vi "UHR-Fleezers Control (host) - 16.2.2v2.vi"() -> ()   [LabVIEW 2014] (continued)
  in  "Limits Enable":bool=TRUE caption="Enable"
  out "AI labels":string[](array[string])=["T1 Y", "T1 X", "T1 Sum", "T2 Y", "T2 X", "T2 Sum", "T1 FB X", "T1 FB Sum", "T2 FB X", "T2 FB Sum", "PSD Y", "PSD X", "PSD Y Sum"]
  in  "Save Trap Pos. Data":bool=TRUE
  in  "Lower Ch. Cap.":bool
  in  "Top 3 Harvard Syringe Pump Serial Port":refnum<visa-resource-name>="Top-Pump3-COM4"
  out "Database link":path
  out "connection reference":T19
  out "FPGA error out":errorcluster
  out "Trigger Signal":dbl[](graph)
  in  "Fish mask thresh":dbl=0.5
  in  "Normal (on) or masked test (off)":bool=TRUE
  in  "Stop F (pN) (mask)":dbl=1.0
  in  "Osc. freq. (Hz)":dbl=0.25
  in  "Trap shift\nmethod":bool=TRUE
  in  "Pause rotation":bool
  out "Waveform Chart":dbl(graph)
  in  "Trap 2 phase shift (deg)":dbl caption="Fixed phase shift (deg)"
  in  "Radius (MHz)":dbl=2.0 min=0.0 max=10.0 step=0.1
  out "Trap trajectories":cluster{dbl[], dbl[]}[](graph)
  in  "Move in a Circle":bool
  in  "Center Y Frequency (MHz)":dbl=31.0
  in  "Stop Moving":bool
  in  "2D Motion Frequency (Hz)":dbl=0.25
  in  "2D Motion Trap Separation (MHz)":dbl=0.75 caption="Fixed distance (MHz)" min=0.0 max=10.0 step=0.1
  in  "Time step (ms)":i64=10
  in  "N steps then stop":i32
  in  "Back to start on finish?":bool=TRUE
  in  "Counterclockwise/Clockwise":bool
  out "Trap 1 sum mean":dbl format="%0.2f"
  out "Trap 2 sum mean":dbl format="%0.2f"
  in  "index 1":i32=3
  in  "index 2":i32
  in  "test":bool
  in  "Reset graph":bool
  in  "N steps to plot":i32=1000
  out "Waveform Graph 2":waveform(dbl)(graph)
  in  "Offset 2":dbl
  in  "mult x":dbl
  in  "Offset":dbl
  out "N data samples":dbl
  out "Initial buffer time (s)":dbl
  in  "N initial buffer elements":u16=5000
  in  "Sound ON":bool
  in  "Carrier Frequency (Hz)":dbl=300.0
  in  "number of samples/ch":i32=100000
  in  "sample mode":T20=1 items=["Finite Samples", "Continuous Samples"]
  in  "device ID":u32
  in  "sound format":T21={"sample rate (S/s)"=22050.0, "number of channels"=2, "bits per sample"=16}
  in  "Volume":dbl=1.0 format="%0.2p"
  in  "interpolation mode":u16(ring)=1 items=["coerce", "linear", "spline", "FIR filter"]
  in  "tone or data":bool
  in  "Data channel to sound":i32
  in  "Base N trap periods":u32=50
  in  "Period scale factor":dbl=4.0
  in  "Trap osc amp (MHz)":dbl=1.0
  in  "Osc trap cont.":bool
  in  "Osc traps":bool
  out "Trap OSC Period (s)":dbl
  out "Writing waveform to fpga memory":bool
  in  "Save trap pos with cal":bool=TRUE
  in  "T1 Osc Enable":bool=TRUE
  in  "T2 Osc Enable":bool=TRUE
  out "DMA remainder":u64
  out "(total save/100) /osc period remainder":u32
  out "Total save/100 remainder":u32
  out "N osc/ (total save/100)":u64
  out "N osc / DMA":u64
  out "N trap osc periods per save":u64
  out "N trap osc periods per save remainder":u64
  in  "Command":string
  out "Reply":string
  in  "Send Command":bool
  out "Preamp Error Out":errorcluster
  in  "Gain Mode":string(combo)="0"
  in  "Invert Signal":bool
  in  "Sensitivity":string(combo)="0"
  in  "Offset Current Sign":bool=TRUE
  in  "Offset Current Value":string(combo)
  in  "Offset Current":bool
  in  "Bias Voltage":bool
  in  "Bias Voltage (mV)":i32
  in  "Filter Type":string(combo)="4"
  in  "Lowpass 3dB Point":string(combo)="6"
  in  "Highpass 3dB Point":string(combo)
  in  "Filter Reset":bool
  out "Command Sent":string
  out "Gain":string(combo)="0"
  # "X"
  # "Y"
  # "APD counting rates"
  # "External fluorescence triggering tests:"
  # "After"
  # "During"
  # "Trap On?"
  # "BD Flow ON?"
  # "Samp Flow ON?"
  # "Trap Trig. Fl.?"
  # "Zero It"
  # "Floor it\n(e.g., hp unwinding)"
  # "1"
  # "2"
  # "Fl. Down"
  # "Fl. Up"
  # "Slowly scan trap from current position to an offset.\nMake range negative to go backwards.\nUses rough Windows timing. \nUpdates trap Delta. \nCan cancel and traps will stay at last position."
  # "Trap Display:"
  # "APD Display:"
  # "Lifetime measurements cannot be make\nat the same time as recording trap positions.\nSo constant force feedback measurements can't be done\n(though constant force can be maintained, just not saved).\nTrap positions also can't be used to do dynamic offset subtraction\n(using the offset curve)."
  # "FPGA DAQ"
  # "Data Saving"
  # "Trap Manipulation"
  # "Bead Calibration"
  # "Fine Motor Control"
  # "Bottom Pump (#1)"
  # "Central Sample Channels"
  # "Top Pump (#3)"
  # "Rate param is ul/h\nVolume param is ul"
  # "Chemyx Pump 2"
  # "Units: \n1 = ml/m\n2 = ml/h\n3 = ul/m\n4 = ul/h"
  # "Some timing delay counts"
  # "Oscillate Set 1 freq. (debugging)"
  # "If using 2nd RF synth board to control green:\nThen small change in FPGA code to make sets 1 and 2\ncorrespond always to board F1 and F2 so green\ndigital out switches between set 1 and 2 frequencies. \nNo third period. \nSet freq for sets 1 and 3 is zero, set 2 is 80 MHz.\nSet amplitude of all three sets to the same value - no feedback yet."
  # "BD 1"
  # "BD 2"
  # "For trap X control"
  # "For green AOM or trap Y control"
  # "Trap interlacing RF phase control"
  # "Phase control methods:\n0 = no phase control\n1 = offset increments each trap cycle by values below\n2 = offset increment increases by increment factor each cycle\n3 = random phase (no parameters to set)"
  # "X"
  # "Y"
  # "Only runs at startup. As of 161102, 30% out gives saturated max AOM out. Amp control is 12 bits, so this max corresponds to ~1300."
  # "14-bit phase number, i.e., 0 to 16383 (2^14) covers full 2*pi phase."
  # "AOD Raster Scan"
  # "Approx. trap separations"
  # "X"
  # "Y"
  # "FPGA\nreading"
  # "DMA\ntransfer"
  # "APD Integration Loop"
  # "APD Gates"
  # "Controls below are for integration occuring right after DMA transfer from FPGA.\nAffects all labview analysis and plotting of fluorescence. \nBUT does not affect data saving. Data is saved at full FPGA integration timing."
  # "APD 2 (Cy5)"
  # "APD 3 (Cy2)"
  # "This needs to be an integer to match trap and fluorescence data transfer timing."
  # "APD 1 (Cy3)"
  # "X"
  # "2D"
  # "Y"
  # "1D"
  # "For producing an anlalog output signal for APDs that can be connected to an oscilloscope and used for alignment within the trap room.\n\nPay attention to FPGA integration time. Needs to be high enough to produce a good signal for each time point. So for a 10 kHz mean fluorescence signal, try 10 ms integration, which would give 100 photons per time point on average."
  # "To switch the excitation laser\nintensity setpoint for each bead pair\n(switches when fishing begins)"
  # "Digital Out Control"
  # "Analog Out Control (Feedback Loop)"
  # "Laser Intensity Analog Input"
  # "Operational note:\n\nUse the digital out control to adjust red laser\ntiming (fine tuning).\n\nAt the moment, the red laser analog out\ncontrol timing is identical and set by green \nlaser AO timing (in the same loop).  Otherwise\nyou can not get synchronous timing with the\ncurrent AO expansion board.\n\nSimilarly, the AI measurement is also \nsimultaneous for all three lasers (for the same\nreason).\n\nThese controls are kept for possible future\nuse."
  # "Analog Out Control (Feedback Loop)"
  # "Digital Out Control"
  # "Laser Intensity Analog Input"
  # "Operational note:\n\nThe AI measurement is simultaneous for all three lasers\n(see red laser note).\n\nThese controls are kept for possible future use."
  # "Analog Out Control (Feedback Loop)"
  # "Laser Intensity Analog Input"
  # "Digital Out Control"
  # "Only initial FIFO depth is set - cannot change while running instrument (will give buffer status error)"
  # "Total AI Rates (NOT rates/trap)"
  # "(Samples/trap x Trap Sets)"
  # "(Samples/channel x\n8 if averaging (8 channels)\n4 if no averaging)"
  # "Trap 1"
  # "Trap 2"
  # "Flour./Trap 3"
  # "External Video Window"
  # "3: IR LED\n2: Blue LED"
  # "MCL Position Debugging"
  # "Temporary Control Storage\n(these used to be somewhere else, still want to keep them)"
  # "Database config"
  # "Y"
  # "X"
  # "Trap Position Difference Limits"
  # "Start trapping above center (> center MHz)\n\nNegative trap separation means trap 2 follows\n(starts to the right)"
  # "Initialization"
  # "Radius initially determined by center\nand current location (then can be changed)"
  # "Active (oscillating) trap calibration:"
  # "All these remainders\nshould be 0."
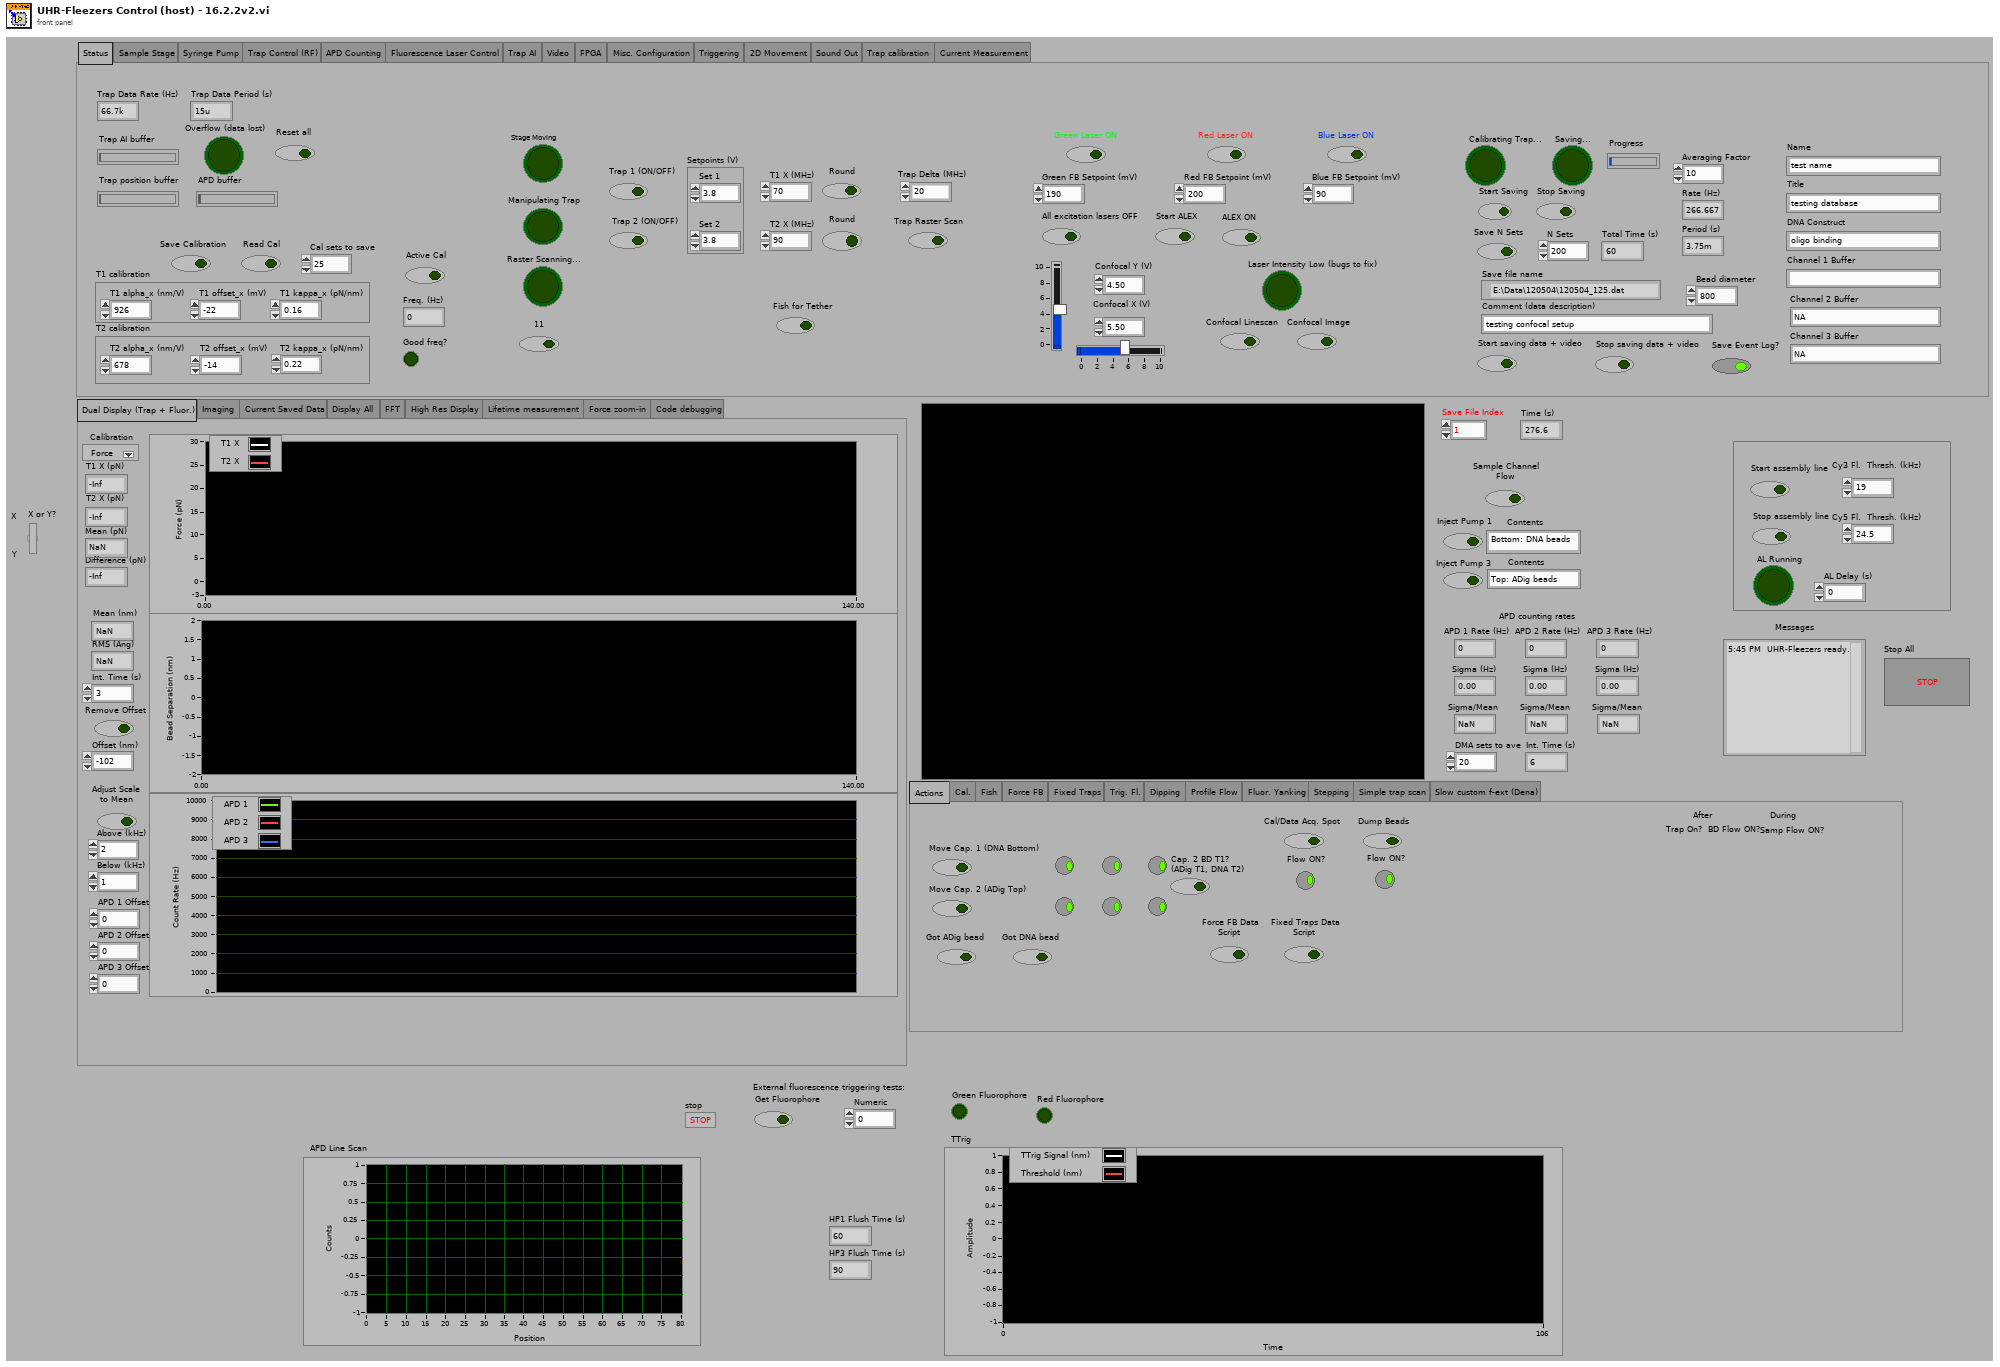
[diagram p1: front panel]
types:
  T1 = enum32{"Actions", "Cal.", "Fish", "Force FB", "Fixed Traps", "Trig. Fl.", "Dipping", "Profile Flow", "Fluor. Yanking", "Stepping", "Simple trap scan", "Slow custom f-ext (Dena)"}
  T2 = typedef "IMAQ Image.ctl" = refnum<image>
  T3 = enum32{"Dual Display (Trap + Fluor.)", "Imaging", "Current Saved Data", "Display All", "FFT", "High Res Display", "Lifetime measurement", "Force zoom-in", "Code debugging"}
  T4 = enum32{"Status", "Sample Stage", "Syringe Pump", "Trap Control (RF)", "APD Counting", "Fluorescence Laser Control", "Trap AI", "Video", "FPGA", "Misc. Configuration", "Triggering", "2D Movement", "Sound Out", "Trap calibration", "Current Measurement"}
  T5 = cluster{"T2 alpha_x (nm/V)":dbl, "T2 offset_x (mV)":dbl, "T2 kappa_x (pN/nm)":dbl}
  T6 = cluster{"T1 alpha_x (nm/V)":dbl, "T1 offset_x (mV)":dbl, "T1 kappa_x (pN/nm)":dbl}
  T7 = cluster{"Pump 1":cluster{"Diameter (mm)":dbl, "Units":dbl, "Volume":dbl, "Rate":dbl}, "Pump 2":cluster{"Diameter (mm)":dbl, "Units":dbl, "Volume":dbl, "Rate":dbl}, "Pump 3":cluster{"Diameter (mm)":dbl, "Units":dbl, "Volume":dbl, "Rate":dbl}}
  T8 = enum32{"IR Laser Interlacing (Direct RF Board Control Method)", "AOD Raster Scan", "Feedback on Trap Intensity", "Feedback on Trap Position"}
  T9 = typedef "LVPoint32TypeDef.ctl" = cluster{"Horizontal":i32, "Vertical":i32}
  T10 = cluster{"Scan Range AOD (nm) 2":dbl, "Step Size AOD (nm) 2":dbl, "Scan Speed AOD (nm/s) 2":dbl, "Number of scans (AOD) 2":u16, "Label":string}[]
  T11 = cluster{"proportional gain (Kc)":i16, "integral gain (Kc*Ts/Ti)":i16, "derivative gain (Kc*Td/Ts)":i16}
  T12 = cluster{"Trap 1":fxp<+/-,16,1>, "Trap 2":fxp<+/-,16,1>}
  T13 = cluster{"proportional gain (Kc)":fxp<+/-,16,8>, "integral gain (Kc*Ts/Ti)":fxp<+/-,16,8>, "derivative gain (Kc*Td/Ts)":fxp<+/-,16,8>}
  T14 = cluster{"output high":fxp<+/-,16,1>, "output low":fxp<+/-,16,1>}
  T15 = cluster{"Set 1":fxp<+/-,16,1>, "Set 2":fxp<+/-,16,1>}
  T16 = enum32{"Main Controls", "Green laser (532 nm)", "Red laser (633 nm)", "Blue laser (473 nm)"}
  T17 = cluster{"Set 1":bool, "Set 2":bool, "Set 3":bool}
  T18 = typedef "LVMinMaxIncTypeDef.ctl" = cluster{"Minimum":dbl, "Maximum":dbl, "Increment":dbl}
  T19 = typedef "NI_Database_API.lvlib/Conn ObjectReference.ctl" = refnum<k1>
  T20 = typedef "Sampling Mode.ctl" = i32
  T21 = typedef "Sound Data Format.ctl" = cluster{"sample rate (S/s)":dbl, "number of channels":i32, "bits per sample":i32}
  T22 = typedef "Image Type" = u32
  T23 = typedef "nirio_resource_hc.ctl" = tag
  T24 = typedef "openfpgaref.initrf.ctl" = refnum<k20>
  T25 = typedef "openfpgaref.8.6.ctl" = refnum<k20>
  T26 = enum16{"empty", "write", "read oldest (queue)", "read newest (stack)", "read all"}
  T27 = cluster{"New Image":T2, "New Image":T2, "New Image":T2, "New Image":T2, "New Image":T2}
  T28 = typedef "XDNodeRunTimeDep.lvlib/timing_clust.ctl" = cluster{"Expected End [f-1]":u64, "Actual End [f-1]":u64, "Finished Late? [f-1]":bool, "Expected End [i-1]":u64, "Actual End [i-1]":u64, "Finished Late? [i-1]":bool, "Expected Start [i]":u64, "Actual Start [i]":u64, "Expected Start [f]":u64, "Actual Start [f]":u64, "Source Name":string, "Structure Name":string, "Period":i64, "Deadline":i64, "Offset":i64, "Start":i64, "Priority":i32, "Timeout":i32, "Mode":T29, "Wakeup Reason":T30, "Error":errorcluster, "Source Type":string, "Secondary Source Type":string, "Global End Time":u64, "Global Start Time":u64, "Frame Duration":u64, "Iteration Duration":u64, "Assigned CPU":i32, "I/O Scan Engine Mode":u32}
  T29 = typedef "XDNodeRunTimeDep.lvlib/nitl_modes.ctl" = enum32{"No Change", "Process missed periods, maintain original phase", "Discard missed periods, maintain original phase", "Process missed periods, ignore original phase", "Discard missed periods, ignore original phase"}
  T30 = typedef "XDNodeRunTimeDep.lvlib/wakeup.ctl" = enum32{"Normal", "Aborted", "Asynchronous wakeup", "Timing source error", "Timed loop error", "Timeout"}
  T31 = enum32{"Status", "Sample Stage", "Syringe Pump", "Trap Control (RF)", "APD Counting", "Fluorescence Laser Control", "Trap AI", "Video", "FPGA"}
  T32 = enum32{"Status", "Sample Stage", "Syringe Pump", "Trap Control (RF)", "APD Counting", "Fluorescence Laser Control", "Trap AI", "Video", "FPGA", "Misc. Configuration"}
  T33 = enum32{"Actions", "Cal.", "Fish", "Force FB", "Fixed Traps", "Trig. Fl.", "Dipping", "Profile Flow", "Fluor. Yanking", "Stepping"}
  T34 = enum16{"big-endian, network order", "native, host order", "little-endian"}
  T35 = enum16{"open", "replace", "create", "open or create", "replace or create", "replace or create with confirmation"}
  T36 = cluster{"Left":i32, "Top":i32, "Width":u32, "Height":u32}
  T37 = cluster{cluster{"Left":i32, "Top":i32, "Width":u32, "Height":u32}}[]
  T38 = cluster{"Scan Range AOD (nm) 2":dbl, "Step Size AOD (nm) 2":dbl, "Scan Speed AOD (nm/s) 2":dbl, "Number of scans (AOD) 2":u16, "Label":string}
  T39 = cluster{"[0]":dbl, "[1]":dbl, "[2]":dbl, "[3]":dbl, "[4]":dbl, "[5]":dbl}
  T40 = cluster{"Diameter (mm)":dbl, "Units":dbl, "Volume":dbl, "Rate":dbl}
  T41 = enum32{"setting", "request", "request control", "info", "statistics", "system settings", "I/O sub system", "HRT control", "camera descriptions", "device specific data", "event sub system settings", "event sub system results", "image memory manager"}
  T42 = typedef "IMAQ AVI2 Refnum.ctl" = refnum<k20>
  T43 = typedef "imagedata.ctl" = cluster{"image type":i32, "image depth":i32, "image":u8[], "mask":u8[], "colors":u32[], "Rectangle":cluster{"left":i16, "top":i16, "right":i16, "bottom":i16}}
  T44 = typedef "Sound Output Task ID.ctl" = u32
  T45 = enum32{"Normal Display", "Dual Display (APD)", "FFT", "High Res Display"}
  T46 = cluster{"Origin Pixel":cluster{"X":sgl, "Y":sgl}, "Angle Relative to Horizontal (deg)":sgl, "Axis Reference":u32}
  T47 = typedef "Simple Grid Descriptor" = cluster{"X Step":sgl, "Y Step":sgl, "Unit":T48}
  T48 = typedef "Image Unit" = enum32{"Undefined", "Angström", "Micrometer", "Millimeter", "Centimeter", "Meter", "Kilometer", "Microinch", "Inch", "Feet", "Nautical miles", "Standard miles", "Steps"}
  T49 = enum32{"Dual Display (Trap + Fluor.)", "Imaging", "Current Saved Data", "Display All", "FFT", "High Res Display"}
  T50 = cluster{"averaging mode":u16, "weighting mode":u16, "number of averages":u32}
  T51 = cluster{"dB On (F)":bool, "unwrap phase (F)":bool, "convert to degree (F)":bool}
  T52 = cluster{"Array Out":dbl[], "Array Out":dbl[], "Array Out":dbl[]}
  T53 = cluster{string, string, string, string, string, string, string, string}
  T54 = cluster{string, string, string, string, string, string, string, string, string, string, string, string}
  T55 = cluster{string, string, string, string, string, string, string, string, string, string, string, string, string}
  T56 = cluster{string, string, string, string, string, string, string, string, string, string, string, string, string, string}
  T57 = cluster{"BD 1 Frequency 1 (MHz)":dbl, "BD 1 Frequency 2 (MHz)":dbl}
  T58 = cluster{"f0":dbl, "df":dbl, "magnitude":dbl[]}[][]
  T59 = cluster{"Comment (data description)":string, "Channel 1 Buffer":string, "Channel 2 Buffer":string, "Channel 3 Buffer":string, "Title":string, "DNA Construct":string, "Bead diameter":dbl, "Name":string}
diagram:
  w7 = u16 20 items=["1.0"=10, "1.5"=15, "2.0"=20] ("stop bits (10: 1 bit)")
  w19 = u16 20 items=["1.0"=10, "1.5"=15, "2.0"=20] ("stop bits (10: 1 bit)")
  w43 = u16 10 items=["1.0"=10, "1.5"=15, "2.0"=20] ("stop bits (10: 1 bit)")
  w56 = u16 20 items=["1.0"=10, "1.5"=15, "2.0"=20] ("stop bits (10: 1 bit)")
  w58 = u16 20 items=["1.0"=10, "1.5"=15, "2.0"=20] ("stop bits (10: 1 bit)")
  w65 = u16 20 items=["1.0"=10, "1.5"=15, "2.0"=20] ("stop bits (10: 1 bit)")
  w48 = T22 2 items=["Grayscale (U8)", "Grayscale (I16)", "Grayscale (SGL)", "Complex (CSG)", "RGB (U32)", "HSL (U32)", "RGB (U64)", "Grayscale (U16)"] ("Image Type")
  # "n samples needed for data"
  # "Settings to help prevent AOM/D damage"
  # "Bottom 1 Harvard"
  # "Top 3 Harvard"
  # "Center Harvard"
  # "Bottom 1 Harvard"
  # "Top 3 Harvard"
  # "Center Harvard"
  n1 = flat-sequence {
    tunnel: [w107] -> w3
    tunnel: [w103] -> w2
    tunnel: w3 -> [w115]
    tunnel: w2 -> [_]
    tunnel: [w110] -> w1
    frame #0 {
      w107 = T23 "750kHzDAQ" ("resource name")
      # "DAQ card ID"
      # "First run the RF synth board initialization fpga code.\n\nThis fpga code essentially enables communication with the RF board using the automatic udclk setting. After running the host initialization vi, the RF boards are fully setup and ready to interlace using the external udclk control. The next fpga code runs the main interlacing instrument methods.\n\nThis host code should run the init bitfile:\n\n'UHR-FleezersInst_FPGATarget_intitializeRFsyn_v1'"
      n2 = xnode "Open FPGA VI Reference"("resource name"=w107) -> ("FPGA VI Reference Out"=w106:refnum<k20>)  [unwired: 1 in, 1 out]
      n3 = xnode "Invoke Method"("FPGA VI Reference In"=w106) -> ("FPGA VI Reference Out"=w100:refnum<k20>, "error out"=w99:errorcluster)  [unwired: 1 in]
      n4 = xnode "Invoke Method"("FPGA VI Reference In"=w100, "error in"=w99) -> ("FPGA VI Reference Out"=w102:refnum<k20>, "error out"=w101:errorcluster)  [unwired: 1 in]
      n5 = call "Initialize RF boards - with FPGA init only vi v1.vi"("error in"=w101, "FPGA Interface"=w102) -> ("error out"=w104:errorcluster, "FPGA Interface 2"=w105:T24)
      n6 = xnode "Close FPGA VI Reference"("FPGA VI Reference In"=w105, "error in"=w104) -> ("error out"=w103:errorcluster)
    }
    frame #1 {
      w108 = TRUE ("PMODE")
      # "Have to set parallel mode and read to high again (they default to low in the FPGA code)"
      # "Then switch to the main fpga code to run the instrument (interlacing fpga code).\n\nThis host code should run the bitfile:\n\n'UHR-FleezersInst_FPGATarget_UHR-Fleezers_main_16.2.1_v3'"
      # "Reset the DAQ card."
      n7 = xnode "Open FPGA VI Reference"("resource name"=w115) -> ("FPGA VI Reference Out"=w114:T25, "error out"=w113:errorcluster)  [unwired: 1 in]
      n8 = xnode "Invoke Method"("FPGA VI Reference In"=w114, "error in"=w113) -> ("FPGA VI Reference Out"=w112:T25, "error out"=w111:errorcluster)
      n9 = xnode "Read/Write Control"("FPGA VI Reference In"=w112, "error in"=w111, "PMODE"=w108, "RD"=w108) -> ("FPGA VI Reference Out"=w110:T25, "error out"=→"FPGA error out":errorcluster)
    }
  }
  n10 = case "Trap X limits" shown="\"1axis\", Default" "1axis AOM vs 2 axis AOD" {
    tunnel: [T18 {"Minimum"=0.0, "Maximum"=40.0, "Increment"=0.1} ("Min Max Inc") T18 {"Minimum"=0.0, "Maximum"=40.0, "Increment"=0.1} ("Min Max Inc") T18 {"Minimum"=0.0, "Maximum"=90.0, "Increment"=1.0} ("Min Max Inc") T18 {"Minimum"=60.0, "Maximum"=90.0, "Increment"=1.0} ("Min Max Inc")] -> w39
    tunnel: [T18 {"Minimum"=0.0, "Maximum"=45.0, "Increment"=1.0} ("Data Entry Limits") T18 {"Minimum"=0.0, "Maximum"=45.0, "Increment"=1.0} ("Data Entry Limits") T18 {"Minimum"=0.0, "Maximum"=50.0, "Increment"=1.0} ("Data Entry Limits") T18 {"Minimum"=0.0, "Maximum"=50.0, "Increment"=1.0} ("Data Entry Limits")] -> w37
    frame "2axisAOD" {
      w117 = u16 300 ("DIO count 1 (ticks)")
      # "Amp Limits"
      # "Freq Limits"
      n11 = disable-structure shown="Disabled" {
        frame Disabled {
          w122 = 35.0 ("BD 1 Amplitude 1 (%)")
          w123 = 30.0 ("BD 1 Frequency 1 (MHz)")
          n12 = local write "BD 1 Frequency 1 (MHz)"(w123) -> ()
          n13 = local write "BD 1 Frequency 2 (MHz)"(w123) -> ()
          n14 = local write "BD 1 Amplitude 2 (%)"(w122) -> ()
          n15 = local write "BD 1 Amplitude 1 (%)"(w122) -> ()
          n16 = local write "BD 2 Frequency 1 (MHz)"(w123) -> ()
          n17 = local write "BD 2 Amplitude 1 (%)"(w122) -> ()
          n18 = local write "BD 2 Frequency 2 (MHz)"(w123) -> ()
          n19 = local write "BD 2 Amplitude 2 (%)"(w122) -> ()
        }
        frame Enabled {
        }
      }
      n20 = local write "All FB On/Off"(FALSE ("All FB On/Off")) -> ()
      n21 = local write "BD 2 Delay (Ticks)"(u8 108 ("BD 2 Delay (Ticks)")) -> ()
      n22 = local write "Number Interlace Sets"(u8 2 ("Number Interlace Sets")) -> ()
      n23 = local write "DIO count 2 (ticks)"(w117) -> ()
      n24 = local write "DIO count 1 (ticks)"(w117) -> ()
    }
    frame "AOD3Sets" {
      w125 = u16 200 ("DIO count 1 (ticks)")
      # "Amp Limits"
      # "Freq Limits"
      n25 = disable-structure shown="Disabled" {
        frame Disabled {
          w130 = 35.0 ("BD 1 Amplitude 1 (%)")
          w131 = 30.0 ("BD 1 Frequency 1 (MHz)")
          n26 = local write "BD 1 Frequency 1 (MHz)"(w131) -> ()
          n27 = local write "BD 1 Frequency 2 (MHz)"(w131) -> ()
          n28 = local write "BD 1 Amplitude 2 (%)"(w130) -> ()
          n29 = local write "BD 1 Amplitude 1 (%)"(w130) -> ()
          n30 = local write "BD 2 Frequency 1 (MHz)"(w131) -> ()
          n31 = local write "BD 2 Amplitude 1 (%)"(w130) -> ()
          n32 = local write "BD 2 Frequency 2 (MHz)"(w131) -> ()
          n33 = local write "BD 2 Amplitude 2 (%)"(w130) -> ()
        }
        frame Enabled {
        }
      }
      n34 = local write "All FB On/Off"(FALSE ("All FB On/Off")) -> ()
      n35 = local write "BD 2 Delay (Ticks)"(u8 0 ("BD 2 Delay (Ticks)")) -> ()
      n36 = local write "Number Interlace Sets"(u8 3 ("Number Interlace Sets")) -> ()
      n37 = local write "DIO count 2 (ticks)"(w125) -> ()
      n38 = local write "DIO count 1 (ticks)"(w125) -> ()
    }
    frame "1axis", Default {
      # "Amp Lmits"
      # "Freq Limits"
    }
    frame "test" {
      # "Amp Lmits"
      # "Freq Limits"
    }
  }
  n39 = flat-sequence "Safety limits on RF frequencies and amplitudes (for AOM protection)" {
    tunnel: [w138] -> w32
    tunnel: [w137] -> w34
    tunnel: [w139] -> w35
    tunnel: [w140] -> w33
    tunnel: w39 -> [w138]
    tunnel: w37 -> [w137]
    tunnel: w1 -> [w136]
    tunnel: [w136] -> w36
    frame #0 {
      w140 = T18 {"Minimum"=0.0, "Maximum"=100.0, "Increment"=0.1} ("Min Max Inc")
      w139 = T18 {"Minimum"=0.0, "Maximum"=35.0, "Increment"=1.0} ("Data Entry Limits")
      n40 = disable-structure shown="Disabled" {
        frame Disabled {
          n41 = property on="BD 1 Frequency 1 (MHz)" class="DigNum (strict)" props=["Data Range"]() -> ()  [unwired: 3 in, 2 out]
          n42 = property on="BD 1 Frequency 2 (MHz)" class="DigNum (strict)" props=["Data Range"]() -> ()  [unwired: 3 in, 2 out]
          n43 = property on="BD 1 Frequency 3 (MHz)" class="DigNum (strict)" props=["Data Range"]() -> ()  [unwired: 3 in, 2 out]
        }
        frame Enabled {
        }
      }
      n44 = property on="BD 2 Frequency 1 (MHz)" class="DigNum (strict)"("Data Range"=w140) -> ()  [unwired: 2 in, 2 out]
      n45 = property on="BD 2 Frequency 3 (MHz)" class="DigNum (strict)"("Data Range"=w140) -> ()  [unwired: 2 in, 2 out]
      n46 = property on="BD 2 Frequency 2 (MHz)" class="DigNum (strict)"("Data Range"=w140) -> ()  [unwired: 2 in, 2 out]
      n47 = property on="BD 2 Amplitude 1 (%)" class="DigNum (strict)"("Data Range"=w139) -> ()  [unwired: 2 in, 2 out]
      n48 = property on="BD 2 Amplitude 2 (%)" class="DigNum (strict)"("Data Range"=w139) -> ()  [unwired: 2 in, 2 out]
      n49 = property on="BD 2 Amplitude 3 (%)" class="DigNum (strict)"("Data Range"=w139) -> ()  [unwired: 2 in, 2 out]
      n50 = property on="BD 1 Amplitude 3 (%)" class="DigNum (strict)"("Data Range"=w137) -> ()  [unwired: 2 in, 2 out]
      n51 = property on="BD 1 Amplitude 2 (%)" class="DigNum (strict)"("Data Range"=w137) -> ()  [unwired: 2 in, 2 out]
      n52 = property on="BD 1 Amplitude 1 (%)" class="DigNum (strict)"("Data Range"=w137) -> ()  [unwired: 2 in, 2 out]
      "X RF Frequency Limits (MHz)" <- w138
      "X RF Amplitude Limits (%)" <- w137
      "Y RF Amplitude Limits (%)" <- w139
      "Y RF Frequency Limits (MHz)" <- w140
    }
  }
  n53 = stacked-sequence "Host initialization sequence - order matters!" {
    tunnel: w36 -> [_ w149 w248 w297 w329 w335 w376 _ w419]
    tunnel: [_ _ _ _ _ _ _ _ w419] -> w16
    tunnel: [_ _ _ _ _ _ _ _ w418] -> w40
    tunnel: w35 -> [_ _ _ _ _ _ w384 _ _]
    tunnel: w34 -> [_ _ _ _ _ _ w383 _ _]
    tunnel: w33 -> [_ _ _ _ _ _ w382 _ _]
    tunnel: w32 -> [_ _ _ _ _ _ w381 _ _]
    frame #0 {
    }
    frame #1 {
      w182 = 10.0 ("y")
      w183 = 32767.0 ("y")
      w167 = 6.0  # clock mult.
      w166 = 49152000.0  # TCXO frequ.
      # "Initialize some FPGA settings"
      n54 = Build Array("DIO count 1 (ticks)", "DIO count 2 (ticks)", "DIO count 3 (ticks)") -> (w217:u16[])
      n55 = local read "AO1"() -> (w188:dbl)
      n56 = local read "AO2"() -> (w189:dbl)
      n57 = local read "Scan Increment (MHz)"() -> (w171:dbl)
      n58 = property on="AI Count (ticks)" class="DigNum (strict)"("Val(Sgnl)"="AI Count (ticks)") -> ()  [unwired: 2 in, 2 out]
      n59 = local read "Continuous MCL Scanning"() -> (w201:bool)
      n60 = local read "Fast Scan Dir"() -> (w202:bool)
      n61 = local read "Number of scans (MCL)"() -> (w200:u64)
      n62 = Multiply(x=w188, y=w183) -> (x*y=w186:dbl)
      n63 = Multiply(x=w189, y=w183) -> (x*y=w184:dbl)
      n64 = Divide(x=40000000.0, y="AI Count (ticks)") -> (x/y=w206:dbl)
      n65 = Divide(x=w186, y=w182) -> (x/y=w187:dbl)
      n66 = Divide(x=w184, y=w182) -> (x/y=w185:dbl)
      n67 = To Word Integer(number=w187) -> (16bit integer=w190:i16)
      n68 = To Word Integer(number=w185) -> (16bit integer=w191:i16)
      n69 = Not(x=w202) -> (.not. x?=w203:bool)
      n70 = local read "Cycles/step (MCL)"() -> (w199:u64)
      n71 = Multiply(x=w171, y=1000.0) -> (x*y=w164:dbl)
      n72 = local read "Scan steps (MCL)"() -> (w198:u64)
      n73 = local write "Trap Pos FIFO Timeout"(u16 0 ("Trap Pos FIFO Timeout")) -> ()
      n74 = local read "Desired Scan Incr (V)"() -> (w196:dbl)
      n75 = local write "AI rate (Hz)"(w206) -> ()
      n76 = Scale By Power Of 2(n=48, x=w164) -> (x*2^n=w163:dbl)
      n77 = Unbundle By Name(cluster{"output high":i16, "output low":i16} {"output high"=3000, "output low"=0} ("FB output range 1")) -> ("output high"=w235:i16, "output low"=w236:i16)
      n78 = Multiply(x=w166, y=w167) -> (x*y=w168:dbl)
      n79 = Divide(x=w163, y=w168) -> (x/y=w169:dbl)
      n80 = local read "Setpoints (V)"() -> (w156:cluster{"Set 1":dbl, "Set 2":dbl})
      n81 = To Quad Integer(1:w169) -> (0:w172:i64)
      n82 = Multiply(x=w196, y=32767.0) -> (x*y=w194:dbl)
      n83 = Divide(x=w206, y="FPGA Ave.") -> (x/y=w205:dbl)
      n84 = local read "Trap Intensity PID Gains"() -> (w161:T11)
      n85 = local read "Next trap write delay (ticks)"() -> (w239:u8)
      n86 = local write "Ave. Rate (Hz)"(w205) -> ()
      n87 = Reciprocal(x=w205) -> (1/x=w204:dbl)
      n88 = local read "Number Interlace Sets"() -> (w224:u8)
      n89 = Split 1D Array(array=w217, index=w224) -> (first subarray=w215:u16[])  [unwired: 1 out]
      n90 = Add Array Elements(numeric array=w215) -> (sum=w216:u16)
      n91 = local write "Ave. Period (s)"(w204) -> ()
      n92 = local read "# Samples/channel"() -> (w179:u32)
      n93 = local read "Number of F/B Scans (AOD)"() -> (w178:u16)
      n94 = local read "Not-Interlacing Set"() -> (w225:enum32{"Set 1", "Set 2", "Set 3"})
      n95 = To Unsigned Byte Integer(number=w225) -> (unsigned 8bit integer=w219:u8)
      n96 = Index Array(array=w217, index=w219) -> (element=w218:u16)
      n97 = local read "Feedback On/Off"() -> (w153:cluster{"Set 1":bool, "Set 2":bool})
      n98 = local read "BD 2 Delay (Ticks)"() -> (w238:u8)
      n99 = local read "BD 1 Delay (ticks)"() -> (w237:u8)
      n100 = local read "Scan steps (AOD)"() -> (w173:u64)
      n101 = local read "All FB On/Off"() -> (w152:bool)
      n102 = local read "Cycles/step (AOD)"() -> (w174:u64)
      n103 = Divide(x=w194, y=10.0) -> (x/y=w195:dbl)
      n104 = Multiply(x=w173, y=w174) -> (x*y=w175:u64)
      n105 = Unbundle By Name(w161) -> ("proportional gain (Kc)"=w231:i16, "integral gain (Kc*Ts/Ti)"=w232:i16, "derivative gain (Kc*Td/Ts)"=w233:i16)
      n106 = Multiply(x=3276.7, y=w156) -> (x*y=w157:cluster{"Set 1":dbl, "Set 2":dbl})
      n107 = To Word Integer(number=w195) -> (16bit integer=w197:i16)
      n108 = Multiply(x=w175, y=u64 2) -> (x*y=w177:u64)
      n109 = To Word Integer(number=w157) -> (16bit integer=w158:cluster{"Set 1":i16, "Set 2":i16})
      n110 = Multiply(x=w177, y=w178) -> (x*y=w180:u64)
      n111 = local read "Sets to FIFO (Traps)"() -> (w228:T17)
      n112 = Divide(x=w180, y=w179) -> (x/y=w181:dbl)
      n113 = Unbundle By Name(w158) -> ("Set 1"=w159:i16, "Set 2"=w160:i16)
      n114 = local read "2D or 1D Scan"() -> (w214:bool)
      n115 = local write "Data points/scans"(w180) -> ()
      n116 = local read "Scan BD"() -> (w162:bool)
      n117 = And(x=w153, y=w152) -> (x .and. y?=w154:cluster{"Set 1":bool, "Set 2":bool})
      n118 = local write "Data points/scan (f/b)"(w177) -> ()
      n119 = local read "N Acq Sets (Traps + Fl.)"() -> (w210:i16)
      n120 = local write "N sets should be saved"(w181) -> ()
      n121 = local read "FPGA error out"() -> (w148:errorcluster)
      n122 = Unbundle By Name(w154) -> ("Set 1"=w150:bool, "Set 2"=w151:bool)
      n123 = local read "Interlace"() -> (w223:bool)
      n124 = Select(t=w216, s=w223, f=w218) -> (s? t:f=w226:u16)
      n125 = local write "Update Count (MCL)"(w226) -> ()
      n126 = local write "Total Counts (ticks)"(w226) -> ()
      n127 = local read "Phase Increment Trap 2"() -> (w141:fxp<+,14,14>)
      n128 = Unbundle By Name(w228) -> ("Set 1"=w229:bool, "Set 2"=w230:bool, "Set 3"=w145:bool)
      n129 = property on="2D or 1D Scan" class="Bool (strict)"("Val(Sgnl)"=w214) -> ()  [unwired: 2 in, 2 out]
      n130 = xnode "Read/Write Control"("FPGA VI Reference In"=w149, "error in"=w148, "ai count"="AI Count (ticks)", "Interlace ON/OFF"=w223, "Number Interlace Cycles"=w224, "Set 1"=w229, "Set 2"=w230, "Set 3"=w145, "RF synth bd controls green"="RF BD 2 to green AOM", "FB On/Off Set 1"=w150, "FB On/Off Set 2"=w151, "Interlace Off Parameters"=w225, "FB Setpoint Set 1"=w159, "FB Setpoint Set 2"=w160, "P1"=w231, "I1"=w232, "D1"=w233, "FB1 output high"=w235, "FB1 output low"=w236, "Cycles per step"=w174, "Scan BD"=w162, "Number of scans"=w178, "Scan steps"=w173, "Scan freq.  increment"=w172, "AO1"=w190, "AO2"=w191, "Scan freq.  increment (MCL)"=w197, "Scan steps (MCL)"=w198, "Cycles per step (MCL)"=w199, "Number of scans (MCL)"=w200, "MCL count"=w226, "Cont. Scan (MCL)"=w201, "MCL Scan Axis"=w203, "1D or 2D Scan?"=w214, "N of AI1 Int Acq Sets"=w210, "Amp switch delay"="RF amplitude switch delay", "Swap F1 and F2"="Swap F1 and F2", "APD to FIFO"=FALSE, "DIO count 1 (ticks)"="DIO count 1 (ticks)", "DIO count 2 (ticks)"="DIO count 2 (ticks)", "DIO count 3 (ticks)"="DIO count 3 (ticks)", "BD 1 Delay (ticks)"=w237, "BD 2 Delay (Ticks)"=w238, "Next trap write delay (ticks)"=w239, "Phase offset method"="Phase offset method", "RF phase reset before cycles"="RF phase reset before cycles", "Phase Trap 1"="Phase Increment Trap 1", "Phase Trap 2"=w141) -> ("error out"=w147:errorcluster)  [unwired: 1 in, 1 out]
      n131 = local write "FPGA error out"(w147) -> ()
    }
    frame #2 {
      # "Initialize some more FPGA settings"
      n132 = local read "Laser interlacing mode"() -> (w249:enum32{"Laser ON", "Laser OFF", "Interlace"})
      n133 = local read "Green Laser ON"() -> (w250:bool)
      n134 = local read "Trap Pos. FB Range"() -> (w271:T14)
      n135 = local read "Trap Pos. FB Gains"() -> (w272:T13)
      n136 = Multiply(x="Green Intensity % (FB OFF)", y=655.35) -> (x*y=w255:dbl)
      n137 = local read "Invert laser interlacing"() -> (w288:bool)
      n138 = local read "Trap Pos. AI1 X Pre-scale"() -> (w265:u16)
      n139 = Multiply(x="Green FB Setpoint (mV)", y=3.2767) -> (x*y=w258:dbl)
      n140 = local read "Trap Pos FB Int Count"() -> (w267:u16)
      n141 = local read "Differential FB?"() -> (w270:bool)
      n142 = local read "Neg. TTrig FPGA"() -> (w268:bool)
      n143 = Multiply(x="Red FB Setpoint (mV)", y=3.2767) -> (x*y=w280:dbl)
      n144 = To Unsigned Word Integer(number=w255) -> (unsigned 16bit integer=w257:u16)
      n145 = Multiply(x="Red Intensity % (FB OFF)", y=655.35) -> (x*y=w284:dbl)
      n146 = To Word Integer(number=w258) -> (16bit integer=w245:i16)
      n147 = Unbundle By Name("Green FB Gains") -> ("proportional gain (Kc)"=w242:i16, "integral gain (Kc*Ts/Ti)"=w241:i16, "derivative gain (Kc*Td/Ts)"=w240:i16)
      n148 = Unbundle By Name("Red FB Gains") -> ("proportional gain (Kc)"=w291:i16, "integral gain (Kc*Ts/Ti)"=w292:i16, "derivative gain (Kc*Td/Ts)"=w293:i16)
      n149 = case shown="False" w250 {
        tunnel: w249 -> [_ w296]
        tunnel: [enum32{"Laser ON", "Laser OFF", "Interlace"}."Laser OFF" ("Green laser mode") w296] -> w289
        frame False {
        }
        frame True {
        }
      }
      n150 = To Word Integer(number=w280) -> (16bit integer=w283:i16)
      n151 = Unbundle By Name(w272) -> ("proportional gain (Kc)"=w276:fxp<+/-,16,8>, "integral gain (Kc*Ts/Ti)"=w277:fxp<+/-,16,8>, "derivative gain (Kc*Td/Ts)"=w278:fxp<+/-,16,8>)
      n152 = To Unsigned Word Integer(number=w284) -> (unsigned 16bit integer=w287:u16)
      n153 = Unbundle By Name(w271) -> ("output high"=w273:fxp<+/-,16,1>, "output low"=w275:fxp<+/-,16,1>)
      n154 = local read "RF BD 2 to green AOM"() -> (w243:bool)
      n155 = local read "Trap Pos FB Monitor\nT1 or T2"() -> (w260:bool)
      n156 = local read "Trap Pos FB Negate Action"() -> (w261:bool)
      n157 = local read "Trap Pos. FB Offset Factor"() -> (w262:i64)
      n158 = local read "Trap Pos. FB Mult Factor"() -> (w263:i64)
      n159 = local read "FPGA error out"() -> (w246:errorcluster)
      n160 = xnode "Read/Write Control"("FPGA VI Reference In"=w248, "error in"=w246, "Invert GI 2"=w288, "Operating Mode 2"=w289, "P3"=w242, "P3 2"=w242, "I3"=w241, "I3 2"=w241, "D3"=w240, "D3 2"=w240, "RF synth bd controls green"=w243, "RF synth green feedback max"="RF synth green feedback max", "Green FB Setpoint 2"=w245, "Green FB Setpoint"=w245, "Green FB On/Off"="Green FB On/Off", "Current Out"=w257, "Green int current ON count adj"="Green int current ON count adj", "Operating Mode"=w289, "Invert GI"=w288, "Trap Pos FB Monitor T1 or T2"=w260, "Trap Pos FB Negate Action"=w261, "Trap Pos. FB Offset Factor"=w262, "Trap Pos. FB Mult Factor"=w263, "Force feedback"=FALSE, "AI1 X Scale"=w265, "Trap Pos to FIFO"=TRUE, "Trap Pos FB Int Count"=w267, "TTrig Negate Pos"=w268, "FB Trig Integrate"="FB Trig Integrate", "Diff FB Measurement?"=w270, "Negate Diff?"="Negate Diff?", "P2"=w276, "I2"=w277, "D2"=w278, "FB2 output high"=w273, "FB2 output low"=w275, "Red FB Setpoint"=w283, "RI Current Out"=w287, "Red Laser Operating Mode"=w289, "RI Operating Mode 2"=w289, "Invert RI 2"=w288, "Invert RI"=w288, "P4"=w291, "I4"=w292, "D4"=w293, "Red FB On/Off"="Red FB On/Off") -> ("error out"=w247:errorcluster)  [unwired: 1 out]
      n161 = local write "FPGA error out"(w247) -> ()
    }
    frame #3 {
      # "Initialize more settings. Should stop using event loops to initialize."
      # "What are these?"
      n162 = stacked-sequence {
        tunnel: w297 -> [_ w311 _ _]
        frame #0 {
          w300 = T26."empty" ("mode")
          # "Clear external fluorescence triggering FIFO"
          # "APD loop counts"
          # "Fluorescence loop counts (rates)"
          n163 = local read "APD Integration Time (s)"() -> (w302:dbl)
          n164 = local read "Interlace ON count"() -> (w303:u16)
          n165 = call "Smart Buffer (DBL) 1.vi"("mode"=w300) -> ()  [unwired: 5 in, 6 out]
          n166 = call "Smart Buffer (DBL) 2.vi"("mode"=w300) -> ()  [unwired: 5 in, 6 out]
          n167 = property on="APD Integration Time (s)" class="DigNum (strict)"("Val(Sgnl)"=w302) -> ()  [unwired: 2 in, 2 out]
          n168 = property on="Interlace ON count" class="DigNum (strict)"("Val(Sgnl)"=w303) -> ()  [unwired: 2 in, 2 out]
          "Number of APDs" <- 3.0 ("Number of APDs")
        }
        frame #1 {
          w309 = 5.0 ("Tick value (ns)")
          # "blue timeout has to start at 0"
          # "Number of APDs affects\nAPD DMA transfer"
          # "General settings for all lasers:"
          # "And includes all laser\nON/OFF settings"
          # "Fluorescent lasers settings:"
          # "Blue laser settings:"
          n169 = local read "ALEX ON"() -> (w312:bool)
          n170 = local read "Lifetime timeout (APD1)"() -> (w304:u16)
          n171 = local read "Laser interlacing mode"() -> (w316:enum32{"Laser ON", "Laser OFF", "Interlace"})
          n172 = local read "Invert laser interlacing"() -> (w315:bool)
          n173 = local read "Blue FB On/Off"() -> (w317:bool)
          n174 = Compound Arithmetic op=MULTIPLY(w304, w309, 0.001 ("Tick value (ns)")) -> (w306:dbl)
          n175 = local write "Lifetime timeout APD1 (us)"(w306) -> ()
          n176 = property on="Blue FB On/Off" class="Bool (strict)"("Val(Sgnl)"=w317) -> ()  [unwired: 2 in, 2 out]
          n177 = xnode "Read/Write Control"("FPGA VI Reference In"=w311, "ALEX green on count"="ALEX green on count", "ALEX red on count"="ALEX red on count", "ALEX ON"=w312, "Lifetime timeout APD1"=0) -> ()  [unwired: 1 in, 2 out]
          n178 = property on="Invert laser interlacing" class="Bool (strict)"("Val(Sgnl)"=w315) -> ()  [unwired: 2 in, 2 out]
          n179 = property on="Laser interlacing mode" class="RadioBtnsControl (strict)"("Val(Sgnl)"=w316) -> ()  [unwired: 2 in, 2 out]
          n180 = local write "Measuring lifetimes"(FALSE ("Measuring lifetimes")) -> ()
          n181 = local write "Trap positions to FIFO"(TRUE ("Trap positions to FIFO")) -> ()
          "Tick value (ns)" <- w309
        }
        frame #2 {
          w318 = path "E:/Home/wheeler/Comstock-LabView-Link.udl" ("connection information")
          # "Initialize the database connection"
          n182 = call-poly <vilib>:"DB Tools Open Connection.vi"("connection information"=w318) -> ("connection reference"=w319:T19)  [unwired: 7 in, 1 out]
          "connection reference" <- w319
          n183 = local write "connection reference"(w319) -> ()
          n184 = local write "Database link"(w318) -> ()
        }
        frame #3 {
          # "Load active calibration to fpga"
          n185 = local read "Base N trap periods"() -> (w321:u32)
          n186 = local read "T1 Osc Enable"() -> (w320:bool)
          n187 = property on="T1 Osc Enable" class="Bool (strict)"("Val(Sgnl)"=w320) -> ()  [unwired: 2 in, 2 out]
          n188 = property on="Base N trap periods" class="DigNum (strict)"("Val(Sgnl)"=w321) -> ()  [unwired: 2 in, 2 out]
        }
      }
      n189 = local write "Offset (nm)"(0.0 ("Offset (nm)")) -> ()
      n190 = local write "Bead Mean (nm)"(0.0 ("Bead Mean (nm)")) -> ()
    }
    frame #4 {
      # "Set FIFO size and run FPGA"
      n191 = local read "FPGA error out"() -> (w328:errorcluster)
      n192 = xnode "Invoke Method"("FPGA VI Reference In"=w329, "error in"=w328, "Requested Depth"="Trap AI FIFO Depth") -> ("FPGA VI Reference Out"=w331:T25, "error out"=w332:errorcluster)  [unwired: 1 out]
      n193 = xnode "Invoke Method"("FPGA VI Reference In"=w331, "error in"=w332, "Requested Depth"="Trap Position FIFO Depth") -> ("FPGA VI Reference Out"=w326:T25, "error out"=w325:errorcluster)  [unwired: 1 out]
      n194 = xnode "Invoke Method"("FPGA VI Reference In"=w326, "error in"=w325, "Requested Depth"="APD FIFO Depth") -> ("FPGA VI Reference Out"=w324:T25, "error out"=w323:errorcluster)  [unwired: 1 out]
      n195 = xnode "Invoke Method"("FPGA VI Reference In"=w324, "error in"=w323) -> ("error out"=w327:errorcluster)  [unwired: 1 in, 1 out]
      n196 = local write "FPGA error out"(w327) -> ()
    }
    frame #5 {
      # "Adjust FPGA timing loop phases"
      n197 = flat-sequence "Initial FPGA Loop Relative Phase Adjustment" {
        tunnel: "Initial Phase Adjustment (AI1)" -> [w366]
        tunnel: "Initial Phase Adjustment (GI)" -> [w365]
        tunnel: "Initial Phase Adj. (MCL)" -> [w364]
        tunnel: [w367] -> w351
        tunnel: [w363] -> w350
        tunnel: "Initial Phase Adjustment (APD Acq)" -> [w362]
        tunnel: "Initial Phase Adjustment (APD 1 Gate)" -> [w361]
        tunnel: "Initial Phase Adjustment (Green FB)" -> [w360]
        tunnel: "Initial Phase Adjustment (GI) 2" -> [w359]
        tunnel: "Initial Phase Adjustment (APD 2 Gate)" -> [w358]
        tunnel: "Initial Phase Adjustment (RI)" -> [w357]
        tunnel: "Initial Phase Adjustment (BI DO)" -> [w356]
        tunnel: "Initial Phase Adjustment (BI AO)" -> [w355]
        tunnel: "Initial Phase Adjustment (APD 3 Gate)" -> [w354]
        tunnel: w335 -> [w353]
        tunnel: w351 -> [w369]
        tunnel: [w370] -> w349
        tunnel: w350 -> [w370]
        tunnel: [w369] -> w348
        tunnel: w349 -> [w374]
        tunnel: w348 -> [w373]
        tunnel: [w371] -> w334
        frame #0 {
          n198 = local read "FPGA error out"() -> (w352:errorcluster)
          n199 = xnode "Read/Write Control"("FPGA VI Reference In"=w353, "error in"=w352, "Phase count adjustment"=w366, "Phase count adjustment (GI)"=w365, "Phase count adjustment (MCL)"=w364, "Phase Count Adjustment (APD Acq)"=w362, "Phase count adjustment (APD 1 Gate)"=w361, "Phase count adjustment (APD 2 Gate)"=w358, "Phase count adjustment (Green FB)"=w360, "Phase count adjustment (GI) 2"=w359, "Phase count adjustment (RI)"=w357, "Phase count adjustment (BI AO)"=w355, "Phase count adjustment (BI D)"=w356, "Phase count adjustment (APD 3 Gate)"=w354) -> ("FPGA VI Reference Out"=w363:T25, "error out"=w367:errorcluster)
        }
        frame #1 {
          n200 = Wait (ms)(milliseconds to wait=u32 100) -> ()  [unwired: 1 out]
        }
        frame #2 {
          w372 = TRUE
          n201 = xnode "Read/Write Control"("FPGA VI Reference In"=w374, "error in"=w373, "+ phase"=w372, "+ phase (GI)"=w372, "+ phase (MCL)"=w372, "+ phase (APD Acq)"=w372, "+ phase (APD 1 Gate)"=w372, "+ phase (APD 2 Gate)"=w372, "+ phase (Green FB)"=w372, "+ phase (GI) 2"=w372, "+ phase (RI)"=w372, "+ phase (BI AO)"=w372, "+ phase (BI D)"=w372, "+ phase (APD 3 Gate)"=w372) -> ("error out"=w371:errorcluster)  [unwired: 1 out]
        }
      }
      n202 = local write "FPGA error out"(w334) -> ()
    }
    frame #6 {
      # "Set RF board initial frequencies and amplitudes"
      n203 = local read "FPGA error out"() -> (w375:errorcluster)
      n204 = call "set RF board frequency - interlace.vi"("Board 2 Frequency Limits"=w382, "Board 1 Frequency Limits"=w381, "error in"=w375, "FPGA VI Reference In"=w376, "Board 2 Frequency 3 (MHz)"="BD 2 Frequency 3 (MHz)", "Board 1 Frequency 3 (MHz)"="BD 1 Frequency 3 (MHz)", "Board 2 Frequency 2 (MHz)"="BD 2 Frequency 2 (MHz)", "Board 2 Frequency 1 (MHz)"="BD 2 Frequency 1 (MHz)", "Board 1 Frequency 2 (MHz)"="BD 1 Frequency 2 (MHz)", "Board 1 Frequency 1  (MHz)"="BD 1 Frequency 1 (MHz)") -> ("error out"=w389:errorcluster, "FPGA VI Reference Out"=w388:T25)
      n205 = call "set RF board amplitude - interlace.vi"("Board 2 Amplitude Limits"=w384, "Board 1 Amplitude Limits"=w383, "error in"=w389, "FPGA VI Reference In"=w388, "Board 2 Amplitude 3 (%)"="BD 2 Amplitude 3 (%)", "Board 1 Amplitude 3 (%)"="BD 1 Amplitude 3 (%)", "Board 2 Amplitude 2 (%)"="BD 2 Amplitude 2 (%)", "Board 2 Amplitude 1 (%)"="BD 2 Amplitude 1 (%)", "Board 1 Amplitude 2 (%)"="BD 1 Amplitude 2 (%)", "Board 1 Amplitude 1 (%)"="BD 1 Amplitude 1 (%)") -> ("error out"=w385:errorcluster)  [unwired: 1 out]
      n206 = local read "Ignore BD 2 for trap delta"() -> (w379:bool)
      n207 = Subtract(x="BD 2 Frequency 1 (MHz)", y="BD 2 Frequency 2 (MHz)") -> (x-y=w397:dbl)
      n208 = Subtract(x="BD 1 Frequency 1 (MHz)", y="BD 1 Frequency 2 (MHz)") -> (x-y=w396:dbl)
      n209 = local write "FPGA error out"(w385) -> ()
      n210 = Square(x=w397) -> (x^2=w380:dbl)
      n211 = Select(t=0.0, s=w379, f=w380) -> (s? t:f=w378:dbl)
      n212 = Square(x=w396) -> (x^2=w398:dbl)
      n213 = Add(x=w398, y=w378) -> (x+y=w399:dbl)
      n214 = Square Root(x=w399) -> (sqrt(x)=w400:dbl)
      n215 = local write "Trap Delta (MHz)"(w400) -> ()
    }
    frame #7 {
      n216 = flat-sequence {
        frame #0 {
          w405 = FALSE ("Retract Pump 3")
          n217 = local read "Trap 1 (ON/OFF)"() -> (w406:bool)
          n218 = local write "Saving..."(FALSE ("Saving Data")) -> ()
          n219 = local write "Stop All"(FALSE ("Stop All")) -> ()
          n220 = local write "Retract Pump 1"(w405) -> ()
          n221 = local write "Retract Pump 3"(w405) -> ()
          n222 = local write "Index"(1.0 ("Index")) -> ()
          n223 = property on="Trap 1 ON" class="Bool (strict)"("Value"=w406) -> ()  [unwired: 2 in, 2 out]
          "Manipulating Trap" <- FALSE ("Manipulating Trap")
        }
        frame #1 {
          n224 = local read "Trap 2 (ON/OFF)"() -> (w411:bool)
          n225 = Wait (ms)(milliseconds to wait=u32 10) -> ()  [unwired: 1 out]
          n226 = property on="Trap 2 ON" class="Bool (strict)"("Val(Sgnl)"=w411) -> ()  [unwired: 2 in, 2 out]
        }
        frame #2 {
          n227 = local read "Scan Range (nm)"() -> (w413:dbl)
          n228 = call "Update messages.vi"("Message to add"="UHR-Fleezers ready.", "Old message string"="") -> ("New message string"=w416:string)
          n229 = local write "Messages"(w416) -> ()
          n230 = property on="Scan Range (nm)" class="DigNum (strict)"("Val(Sgnl)"=w413) -> ()  [unwired: 2 in, 2 out]
        }
      }
    }
    frame #8 {
      # "Wait 5 s for all the event loops still being executed to finish."
      n231 = Wait (ms)(milliseconds to wait=u32 5000) -> ()  [unwired: 1 out]
      n232 = local read "FPGA error out"() -> (w418:errorcluster)
    }
  }
  n233 = call-poly "VISA Configure Serial Port"("VISA resource name"=refnum<visa-resource-name> "COM2", "baud rate (9600)"=u32 9600, "stop bits (10: 1 bit)"=w19) -> ("VISA resource name out"=w8:refnum<visa-resource-name>, "error out"=→"Preamp Error Out":errorcluster)  [unwired: 4 in, 7 out]
  n234 = call-poly "VISA Configure Serial Port"("VISA resource name"=refnum<visa-resource-name> "COM2", "baud rate (9600)"=u32 9600, "stop bits (10: 1 bit)"=w7) -> ("VISA resource name out"=w5:refnum<visa-resource-name>)  [unwired: 4 in, 8 out]
  n235 = call-poly "VISA Configure Serial Port"("VISA resource name"=refnum<visa-resource-name> "COM7", "baud rate (9600)"=u32 115200, "stop bits (10: 1 bit)"=w43) -> ("VISA resource name out"=w42:refnum<visa-resource-name>, "error out"=w41:errorcluster)  [unwired: 4 in, 7 out]
  n236 = local write "Blue Error Out"(w41) -> ()
  n237 = call-poly "VISA Configure Serial Port"("VISA resource name"=refnum<visa-resource-name> "COM5", "baud rate (9600)"=u32 115200, "stop bits (10: 1 bit)"=w56) -> ("VISA resource name out"=w53:refnum<visa-resource-name>, "error out"=w52:errorcluster)  [unwired: 4 in, 7 out]
  n238 = call-poly "VISA Configure Serial Port"("VISA resource name"=refnum<visa-resource-name> "COM4", "baud rate (9600)"=u32 115200, "stop bits (10: 1 bit)"=w58) -> ("VISA resource name out"=w55:refnum<visa-resource-name>, "error out"=w54:errorcluster)  [unwired: 4 in, 7 out]
